vi "niFpgaFFTCore.vi"(0 "real data in":fxp<+/-,16,1> format="%#.16g", 1 "reset":bool, 5 "imaginary data in":fxp<+/-,16,1> format="%#.16g", 7 "input valid":bool=TRUE, 12 "ready for output":bool=TRUE) -> (3 "data index":u16, 4 "real data out":fxp<+/-,16,12> format="%.8g", 6 "imaginary data out":fxp<+/-,16,12> format="%.8g", 8 "output valid":bool, 14 "ready for input":bool)   [LabVIEW 2017]
uses:
  <vilib>/rvi/LocalResourceManager/LocalResourceManager.xnode
  <vilib>/rvi/FXPMathLib/basic elements/FxpDiscreteDelay/XNode/nifxpmath_DiscreteDelay.xnode
  <vilib>/rvi/DataTransferAndStorage/Container/XNode/niFpgaContainer.xnode
  <vilib>/rvi/Memory/Memory_Emulation/niFpgaMemoryEmulationRefIn.vi
  <vilib>/rvi/DataTransferAndStorage/Container/Common/niFpgaContainerGetUniqueNameForEmu.vi
  <vilib>/rvi/DataTransferAndStorage/Container/Common/niFpgaContainerSetEmuInfo.vi
  <vilib>/rvi/eio/common/nirviEmuReportErrorAndStop.vi
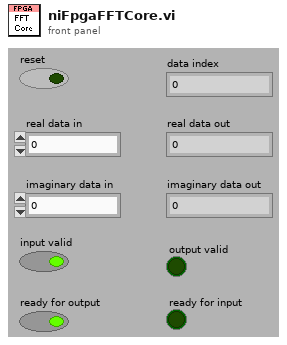
[diagram p1: front panel]
types:
  T1 = cluster{"N/2-1":u16, "(N/2)*K + 2":u16, "(N/2)*(K-1)+2":u16, "(N/2)*K + 1 + N/2":u16, "N-1":u16, "total latency":u16, "K - 1":u8, "K - 16":i8, "K - 17":i8}
  T2 = cluster{"Real":fxp<+/-,16,1>, "Imaginary":fxp<+/-,16,1>}
  T3 = typedef "niFPGA FFT Control Signals.ctl" = cluster{"read address":u16, "switch":bool, "write input to B":bool, "write stage results":bool, "write input to A":bool, "output valid":bool, "twiddle address":u16, "write address":u16, "outputs from mem":bool, "ready for data":bool, "stage":u8}
  T4 = cluster{"addr":u16, "enable":bool, "data":cluster{"Real":fxp<+/-,16,1>, "Imaginary":fxp<+/-,16,1>}}
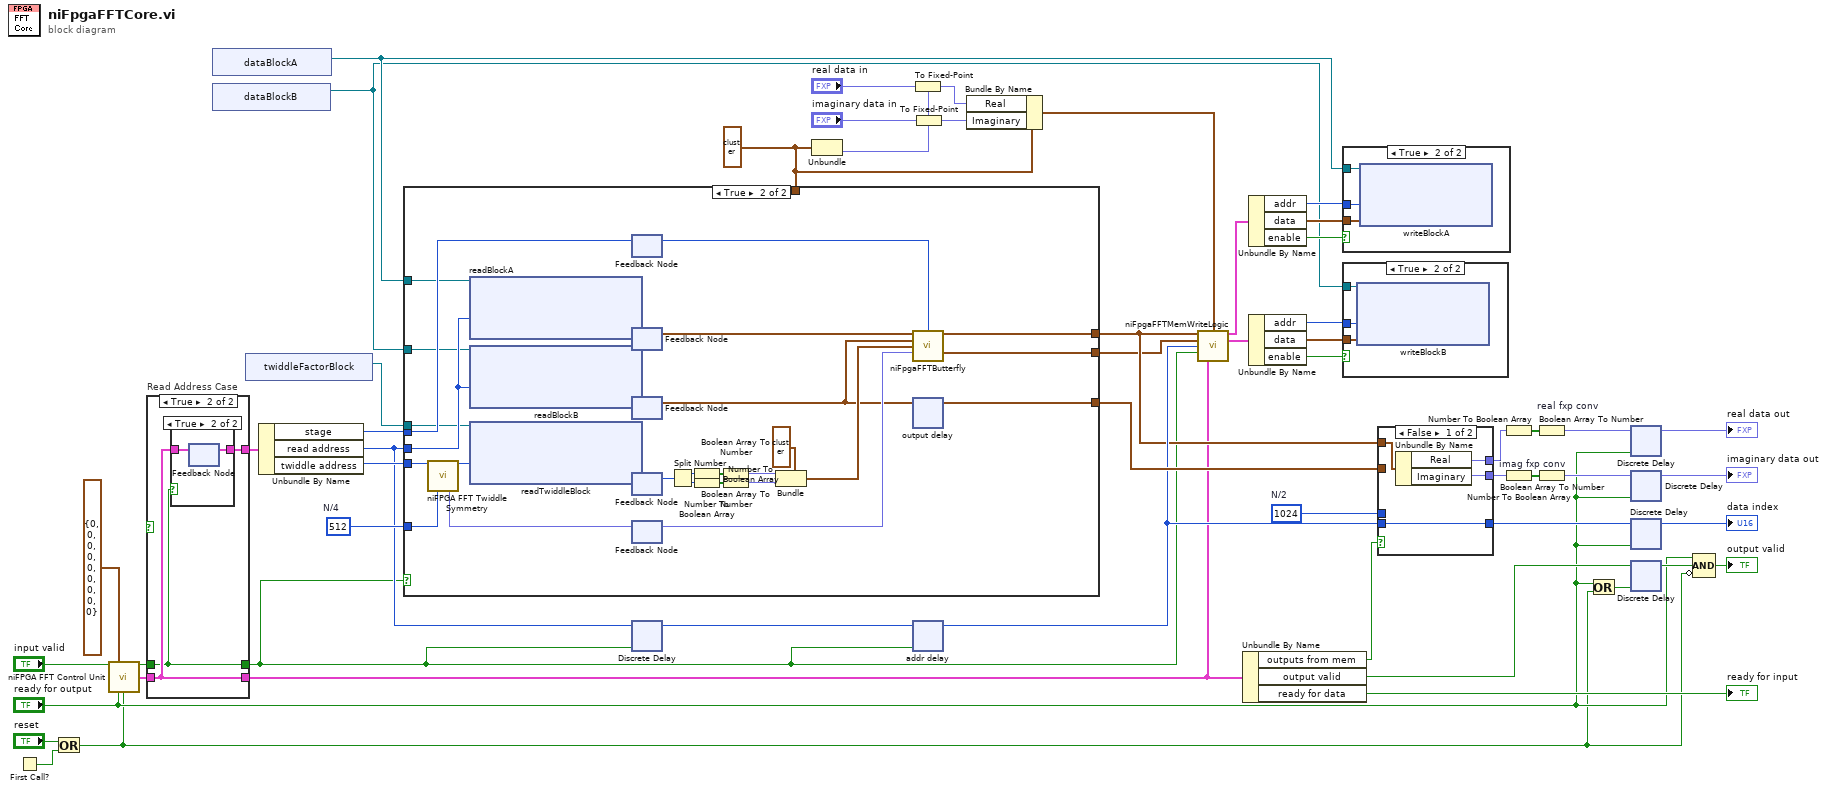
[diagram p0: block diagram]
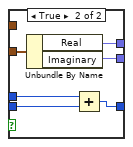
[diagram p4: hidden frame]
diagram:
  w33 = u16 1024  # N/2
  w37 = u16 512  # N/4
  w41 = T2 {"Real"=0.0, "Imaginary"=0.0} ("internalComplexType")
  n1 = First Call?() -> (First Call?: T/F=w13:bool)
  n2 = Or(x="reset", y=w13) -> (x .or. y?=w9:bool)
  n3 = call <vilib>:"niFPGA FFT Control Unit.vi"("input valid"="input valid", "Execution Constants"=T1 {"N/2-1"=0, "(N/2)*K + 2"=0, "(N/2)*(K-1)+2"=0, "(N/2)*K + 1 + N/2"=0, "N-1"=0, "total latency"=0, "K - 1"=0, "K - 16"=0, "K - 17"=0}, "ready for output"="ready for output", "reset"=w9) -> ("enable fft"=w6:bool, "control signals out"=w7:T3)  [unwired: 10 in]
  n4 = case "Read Address Case" shown="True" {
    selector: _ -> [_ _]
    tunnel: w7 -> [w57 w59]
    tunnel: [w57 w60] -> w8
    tunnel: w6 -> [w56 w58]
    tunnel: [w56 w58] -> w5
    tunnel: [w57 w59] -> w4
    frame False {
    }
    frame True {
      n5 = case shown="True" w58 {
        tunnel: [_ w62] -> w60
        tunnel: w59 -> [_ w61]
        frame False {
        }
        frame True {
          n6 = feedback-in #1(w61) -> ()
          n7 = feedback #1() -> (w62:T3)  [unwired: 1 in]
        }
      }
    }
  }
  n8 = xnode ("dataBlockA")() -> ("Memory Out"=w2:refnum<k21>)
  n9 = xnode ("dataBlockB")() -> ("Memory Out"=w1:refnum<k21>)
  n10 = xnode ("twiddleFactorBlock")() -> ("Memory Out"=w3:refnum<k21>)
  n11 = Unbundle By Name(w8) -> ("stage"=w14:u8, "read address"=w32:u16, "twiddle address"=w45:u16)
  n12 = case shown="True" w5 {
    tunnel: w45 -> [_ w74]
    tunnel: [_ w69] -> w28
    tunnel: [_ w90] -> w29
    tunnel: w41 -> [_ _]
    tunnel: w14 -> [_ w78]
    tunnel: w37 -> [_ w82]
    tunnel: [_ w68] -> w34
    tunnel: w32 -> [_ w83]
    tunnel: w2 -> [_ w65]
    tunnel: w1 -> [_ w64]
    tunnel: w3 -> [_ w63]
    frame False {
    }
    frame True {
      n13 = call <vilib>:"niFPGA FFT Twiddle Symmetry.vi"("twiddle index"=w74, "N/4"=w82) -> ("modified twiddle index"=w73:u16, "flag"=w71:fxp<+,2,2>)  [unwired: 12 in]
      n14 = xnode ("readBlockA")("Address"=w83, "Memory In"=w65) -> ("Data"=w79:T2)  [unwired: 1 out]
      n15 = xnode ("readBlockB")("Address"=w83, "Memory In"=w64) -> ("Data"=w80:T2)  [unwired: 1 out]
      n16 = xnode ("readTwiddleBlock")("Address"=w73, "Memory In"=w63) -> ("Data"=w81:u32)  [unwired: 1 out]
      n17 = feedback-in #2(w78) -> ()
      n18 = feedback #2() -> (w76:u8)  [unwired: 1 in]
      n19 = feedback-in #3(w79) -> ()
      n20 = feedback #3() -> (w67:T2)  [unwired: 1 in]
      n21 = feedback-in #4(w80) -> ()
      n22 = feedback #4() -> (w66:T2)  [unwired: 1 in]
      n23 = feedback-in #5(w81) -> ()
      n24 = feedback #5() -> (w77:u32)  [unwired: 1 in]
      n25 = feedback-in #6(w71) -> ()
      n26 = feedback #6() -> (w70:fxp<+,2,2>)  [unwired: 1 in]
      n27 = Split Number(x=w77) -> (hi(x)=w84:u16, lo(x)=w86:u16)
      n28 = Number To Boolean Array(number=w84) -> (Boolean array=w89:bool[])
      n29 = Number To Boolean Array(number=w86) -> (Boolean array=w88:bool[])
      n30 = Boolean Array To Number ("fxpForCluster7")(Boolean array=w89) -> (number=w72:fxp<+/-,16,1>)
      n31 = Boolean Array To Number ("fxpForCluster8")(Boolean array=w88) -> (number=w87:fxp<+/-,16,1>)
      n32 = Bundle(cluster=T2 {"Real"=0.0, "Imaginary"=0.0} ("internalTwiddleType"), "Real"=w72, "Imaginary"=w87) -> (w75:T2)
      n33 = call <vilib>:"niFpgaFFTButterfly.vi"("X in"=w67, "stage"=w76, "Y in"=w66, "TwiddleFactor"=w75, "flag"=w70) -> ("X out"=w90:T2, "Y out"=w69:T2)  [unwired: 9 in]
      n34 = xnode "output delay"("D"=w66) -> ("Q"=w68:T2)
    }
  }
  n35 = xnode ("Discrete Delay")("D"=w32, "enable"=w5) -> ("Q"=w26:u16)
  n36 = Unbundle(w41) -> ("Imaginary"=w40:fxp<+/-,16,1>)  [unwired: 1 out]
  n37 = To Fixed-Point(fixed-point type=w40, number="real data in") -> (fixed-point=w39:fxp<+/-,16,1>)
  n38 = xnode "addr delay"("D"=w26, "enable"=w5) -> ("Q"=w30:u16)
  n39 = To Fixed-Point(fixed-point type=w40, number="imaginary data in") -> (fixed-point=w42:fxp<+/-,16,1>)
  n40 = Bundle By Name(cluster=w41, "Real"=w39, "Imaginary"=w42) -> (w31:T2)
  n41 = call <vilib>:"niFpgaFFTMemWriteLogic.vi"("x from bf"=w29, "input data"=w31, "y from bf"=w28, "read address"=w30, "enable mem"=w5, "control signals"=w4) -> ("memory output A"=w49:T4, "memory output B"=w48:T4)  [unwired: 8 in]
  n42 = Unbundle By Name(w4) -> ("outputs from mem"=w27:bool, "output valid"=w15:bool, "ready for data"=→"ready for input":bool)
  n43 = Unbundle By Name(w49) -> ("addr"=w50:u16, "data"=w51:T2, "enable"=w52:bool)
  n44 = Unbundle By Name(w48) -> ("addr"=w55:u16, "data"=w54:T2, "enable"=w53:bool)
  n45 = case shown="True" w52 {
    tunnel: w51 -> [_ w93]
    tunnel: w50 -> [_ w92]
    tunnel: w2 -> [_ w91]
    frame False {
    }
    frame True {
      n46 = xnode ("writeBlockA")("Address"=w92, "Data"=w93, "Memory In"=w91) -> ()  [unwired: 1 in, 2 out]
    }
  }
  n47 = case shown="True" w53 {
    tunnel: w55 -> [_ w96]
    tunnel: w54 -> [_ w95]
    tunnel: w1 -> [_ w94]
    frame False {
    }
    frame True {
      n48 = xnode ("writeBlockB")("Address"=w96, "Data"=w95, "Memory In"=w94) -> ()  [unwired: 1 out]
    }
  }
  n49 = case shown="False" w27 {
    tunnel: w29 -> [w100 _]
    tunnel: [w99 w106] -> w36
    tunnel: [w98 w105] -> w35
    tunnel: w34 -> [_ w104]
    tunnel: w30 -> [w97 w103]
    tunnel: [w97 w102] -> w20
    tunnel: w33 -> [_ w101]
    frame False {
      n50 = Unbundle By Name(w100) -> ("Real"=w99:fxp<+/-,16,1>, "Imaginary"=w98:fxp<+/-,16,1>)
    }
    frame True {
      n51 = Unbundle By Name(w104) -> ("Real"=w106:fxp<+/-,16,1>, "Imaginary"=w105:fxp<+/-,16,1>)
      n52 = Add(x=w101, y=w103) -> (x+y=w102:u16)
    }
  }
  n53 = Number To Boolean Array(number=w36) -> (Boolean array=w46:bool[])
  n54 = Number To Boolean Array(number=w35) -> (Boolean array=w47:bool[])
  n55 = Boolean Array To Number "real fxp conv"(Boolean array=w46) -> (number=w21:fxp<+/-,16,12>)
  n56 = Boolean Array To Number "imag fxp conv"(Boolean array=w47) -> (number=w24:fxp<+/-,16,12>)
  n57 = Or(x="ready for output", y=w9) -> (x .or. y?=w10:bool)
  n58 = xnode ("Discrete Delay")("D"=w21, "enable"="ready for output") -> ("Q"=→"real data out":fxp<+/-,16,12>)
  n59 = xnode ("Discrete Delay")("D"=w24, "enable"="ready for output") -> ("Q"=→"imaginary data out":fxp<+/-,16,12>)
  n60 = xnode ("Discrete Delay")("D"=w20, "enable"="ready for output") -> ("Q"=→"data index":u16)
  n61 = xnode ("Discrete Delay")("D"=w15, "enable"=w10) -> ("Q"=w25:bool)
  n62 = Compound Arithmetic op=AND("ready for output", w25, invert w9) -> (→"output valid":bool)
